vi "Filter Data.vi"(8 "error in (no error)":errorcluster, 10 "Debug Data In":refnum<class "Debug Data.lvclass">[](array[class]), 11 "Filter by Process in":refnum<class "Filter by Is Receive.lvclass">) -> (0 "error out":errorcluster, 2 "Debug Data Out":refnum<class "Debug Data.lvclass">[](array[class]), 3 "Filter by Process out":refnum<class "Filter by Is Receive.lvclass">)   [LabVIEW 2020, in "Filter by Is Receive.lvclass"]
uses:
  Filter by Is Receive.lvclass
  Debug Data/Debug Data.lvclass
  Filter by Is Receive.lvclass/Filter by Is Receive.ctl
  Debug Data/Debug Data.lvclass/Debug Data.ctl
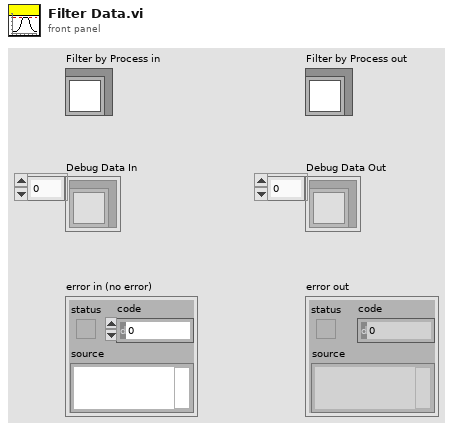
[diagram p1: front panel]
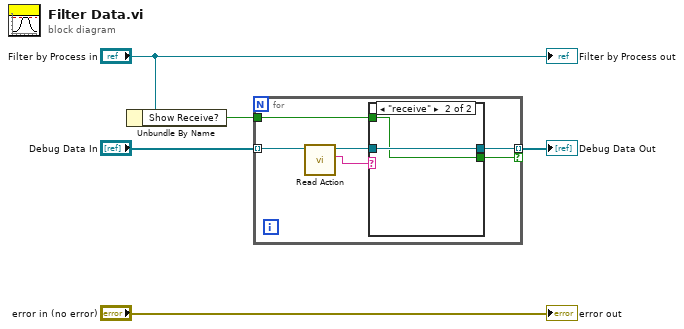
[diagram p0: block diagram]
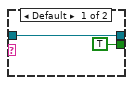
[diagram p2: hidden frame]
diagram:
  n1 = Unbundle By Name("Filter by Process in") -> ("Show Receive?"=w1:bool)
  n2 = for {
    tunnel: [w9] -> w3 mode=indexing if=w7
    tunnel: "Debug Data In" -> [w11] mode=indexing
    tunnel: w1 -> [w6]
    n3 = call "Read Action.vi"("Debug Data in"=w11) -> ("Action"=w10:string, "Debug Data out"=w8:refnum<class "Debug Data.lvclass">)  [unwired: 8 in, 1 out]
    n4 = case shown="\"receive\"" w10 {
      tunnel: [w13 w15] -> w9
      tunnel: w8 -> [w13 w15]
      tunnel: [TRUE ("Show Send?") w14] -> w7
      tunnel: w6 -> [_ w14]
      frame Default {
      }
      frame "receive" {
      }
    }
  }
  "Debug Data Out" <- w3
  "error out" <- "error in (no error)"
  "Filter by Process out" <- "Filter by Process in"
